vi "Register Open Handle.vi"(8 "error in":errorcluster, 10 "handle":T1 format="%02x", 11 "session in":refnum<class "Session.lvclass">) -> (0 "error out":errorcluster, 3 "session out":refnum<class "Session.lvclass">)   [LabVIEW 2020, in "NI_SFTP.lvlib" / "Session.lvclass"]
uses:
  <vilib>/net/SFTP/Session/Session.lvclass
  <vilib>/net/SFTP/Session/Handle.ctl
  <vilib>/net/SFTP/Session/Session.lvclass/Session.ctl
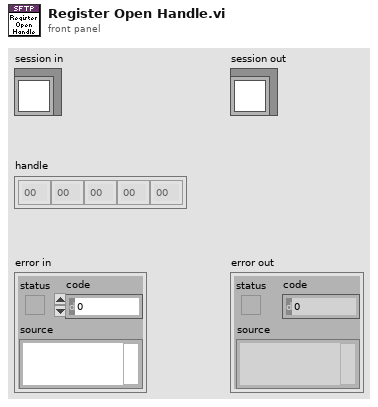
[diagram p1: front panel]
types:
  T1 = typedef "NI_SFTP.lvlib/Session.lvclass/Handle.ctl" = u8[]
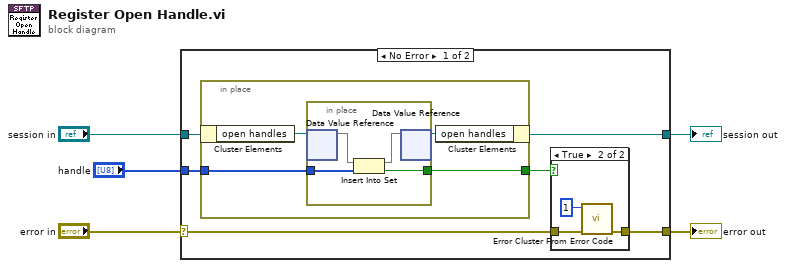
[diagram p0: block diagram]
diagram:
  n1 = case shown="No Error" "error in" {
    selector: "error in" -> [w7 w25]
    tunnel: [w6 w25] -> w4
    tunnel: [w9 w24] -> w2
    tunnel: "session in" -> [w11 w24]
    tunnel: "handle" -> [w10 _]
    frame No Error {
      n2 = in-place {
        in-place-border: w10 -> [w18]
        in-place-border: [w16] -> w8
        n3 = in-place-cluster #1(w11) -> ("open handles"=w19:refnum<data-value>)
        n4 = in-place {
          in-place-border: w18 -> [w22]
          in-place-border: [w20] -> w16
          n5 = in-place-dvr #2(w19) -> (w23:set{T1})  [unwired: 1 out]
          n6 = Insert Into Set(10:w22, 11:w23) -> (2:w20:bool, 3:w21:set{T1})
          n7 = in-place-dvr #2(w21) -> (w17:refnum<data-value>)  [unwired: 1 out]
        }
        n8 = in-place-cluster #1("open handles"=w17) -> (w9:refnum<class "Session.lvclass">)
      }
      n9 = case shown="True" w8 {
        tunnel: w7 -> [w12 w15]
        tunnel: [w12 w14] -> w6
        frame False {
        }
        frame True {
          n10 = call <vilib>:"Error Cluster From Error Code.vi"("error in (no error)"=w15, "error code (0)"=1) -> ("error out"=w14:errorcluster)  [unwired: 7 in]
        }
      }
    }
    frame Error {
    }
  }
  "error out" <- w4
  "session out" <- w2
